vi "readFromXML.vi"(8 "error in (no error)":errorcluster, 10 "XML in":string="<GuiderName>\n  <guiderName>isSHMES</guiderName>\n</GuiderName>", 11 "GuiderName in":refnum<class "GuiderName.lvclass">) -> (0 "error out":errorcluster, 3 "GuiderName out":refnum<class "GuiderName.lvclass">)   [LabVIEW 2014, in "TCSDataDefinitions.lvlib" / "TCSGuiderCommand.lvlib" / "GuiderName.lvclass"]
uses:
  GuiderName.lvclass
  GuiderName.lvclass/GuiderName.ctl
  TCSGuiderCommand/TCSGuiderCommand.lvclass
  <userlib>/Common/XML/XMLParser/XMLParser.lvclass
panel:
  out "string":string="isSHMES"
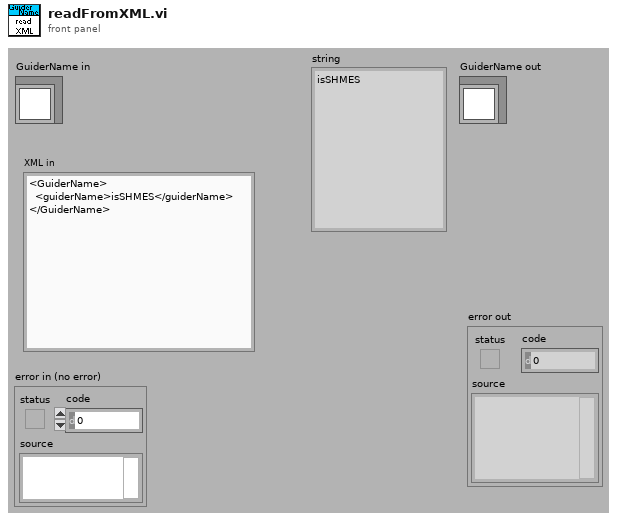
[diagram p1: front panel]
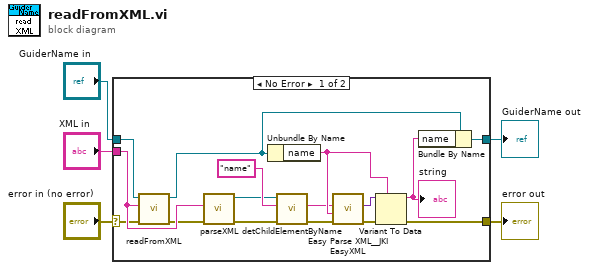
[diagram p0: block diagram]
diagram:
  n1 = case shown="No Error" "error in (no error)" {
    selector: "error in (no error)" -> [w12 w23]
    tunnel: [w16 w23] -> w4
    tunnel: [w17 w22] -> w2
    tunnel: "GuiderName in" -> [w15 w22]
    tunnel: "XML in" -> [w13 _]
    frame No Error {
      n2 = call-parent "readFromXML.vi"("error in (no error)"=w12, "XML in"=w13, "TCSGuiderCommand.lvclass"=w15) -> ("error out"=w11:errorcluster, "TCSGuiderCommand.lvclass 2"=w14:refnum<class "GuiderName.lvclass">)  [unwired: 7 out]
      n3 = call <userlib>:"parseXML.vi"("error in (no error)"=w11, "XMLString in"=w13) -> ("error out"=w7:errorcluster, "Element out"=w6:refnum<class "XMLParser.lvclass">)  [unwired: 8 in]
      n4 = Unbundle By Name(w14) -> ("name"=w19:string)
      n5 = call <userlib>:"detChildElementByName.vi"("error in (no error)"=w7, "childName"="name" ("ChildName"), "Element in"=w6) -> ("error out"=w8:errorcluster, "childXML"=w9:string)  [unwired: 5 in, 2 out]
      n6 = call <vilib>:"Easy Parse XML__JKI EasyXML.vi"("error in (no error)"=w8, "LabVIEW Data (Type)"=w19, "XML String"=w9) -> ("error out"=w21:errorcluster, "LabVIEW Data"=w20:variant)  [unwired: 7 out]
      n7 = Variant To Data(error in=w21, type=w19, Variant=w20) -> (data=w18:string, error out=w16:errorcluster)
      "string" <- w18
      n8 = Bundle By Name(cluster=w14, "name"=w18) -> (w17:refnum<class "GuiderName.lvclass">)
    }
    frame Error {
    }
  }
  "error out" <- w4
  "GuiderName out" <- w2
